vi "read_acq_mode.vi"(8 "error in (no error)":errorcluster, 11 "detector in":refnum<class "detector.lvclass">) -> (0 "error out":errorcluster, 2 "Mode":T1 items=["T2"=2, "T3"=3], 3 "detector out":refnum<class "detector.lvclass">)   [LabVIEW 2015, in "detector.lvclass"]
uses:
  detector.lvclass
  Picoquant/Hydraharp/hydraharp_panel/hpanel_acq_modes.ctl
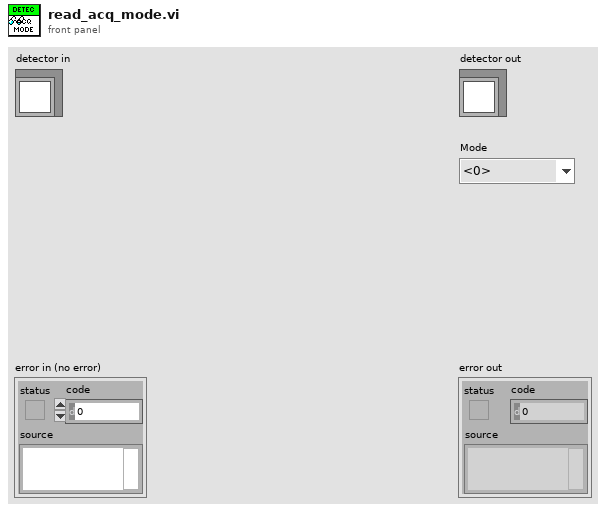
[diagram p1: front panel]
types:
  T1 = typedef "hpanel_acq_modes.ctl" = u16
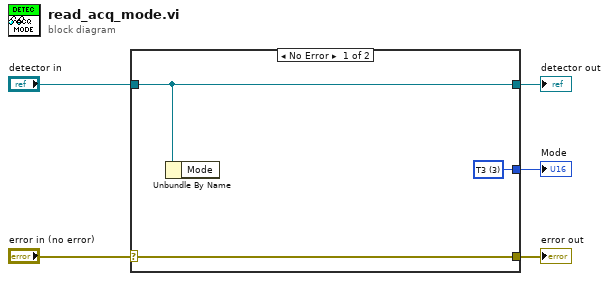
[diagram p0: block diagram]
diagram:
  n1 = case shown="No Error" "error in (no error)" {
    selector: "error in (no error)" -> [w8 w9]
    tunnel: [w8 w9] -> w4
    tunnel: [w7 w10] -> w2
    tunnel: "detector in" -> [w7 w10]
    tunnel: [w6 _] -> w1
    frame No Error {
      w6 = T1 3 items=["T2"=2, "T3"=3] ("Mode")
      n2 = Unbundle By Name(w7) -> ()  [unwired: 1 out]
    }
    frame Error {
    }
  }
  "error out" <- w4
  "detector out" <- w2
  "Mode" <- w1
